vi "Test Cryostat API.vi"   [LabVIEW 2016, in "Instrument.Cryostat.lvclass"]
uses:
  Instrument.Cryostat.lvclass
  <vilib>/addons/_JKI Toolkits/Caraya/classes/Test/Test.lvclass
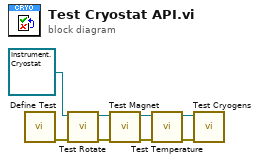
[diagram p0: block diagram]
diagram:
  n1 = call <vilib>:"Define Test.vi"() -> ("error out"=w3:errorcluster)  [unwired: 11 in]
  n2 = call "Test Rotate.vi"("error in (no error)"=w3, "Instrument.Cryostat in"=refnum<class "Instrument.Cryostat.lvclass"> refnum) -> ("error out"=w7:errorcluster, "Instrument.Cryostat out"=w5:refnum<class "Instrument.Cryostat.lvclass">)  [unwired: 8 in]
  n3 = call "Test Magnet.vi"("error in (no error)"=w7, "Instrument.Cryostat in"=w5) -> ("error out"=w2:errorcluster, "Instrument.Cryostat out"=w6:refnum<class "Instrument.Cryostat.lvclass">)  [unwired: 8 in]
  n4 = call "Test Temperature.vi"("error in (no error)"=w2, "Instrument.Cryostat in"=w6) -> ("error out"=w1:errorcluster, "Instrument.Cryostat out"=w4:refnum<class "Instrument.Cryostat.lvclass">)  [unwired: 8 in]
  n5 = call "Test Cryogens.vi"("error in (no error)"=w1, "Instrument.Cryostat in"=w4) -> ()  [unwired: 8 in, 2 out]
